vi "fuzzyex Set Move Direction.vi"(1 "方向":bool, 2 "beta":dbl format="%.2f", 3 "y(VC)":dbl format="%.2f", 4 "x(VC)":dbl format="%.2f") -> (0 "新建目录":bool)   [LabVIEW 2018]
doc: "本VI根据车辆中心坐标、车辆方位角和当前移动方向，在车辆驱动控制范例中计算适当的移动方向。如果车辆不能向后移动到其最终位置，则前进，获得足够的空间后再后退。"
panel:
  # "车辆中心的X坐标"
  # "前进行驶"
  # "车辆中心的Y坐标"
  # "后退行驶"
  # "车辆方位角"
  # "前进行驶"
  # "后退行驶"
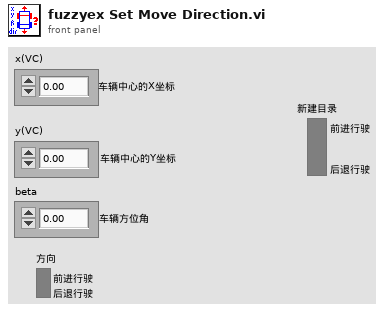
[diagram p1: front panel]
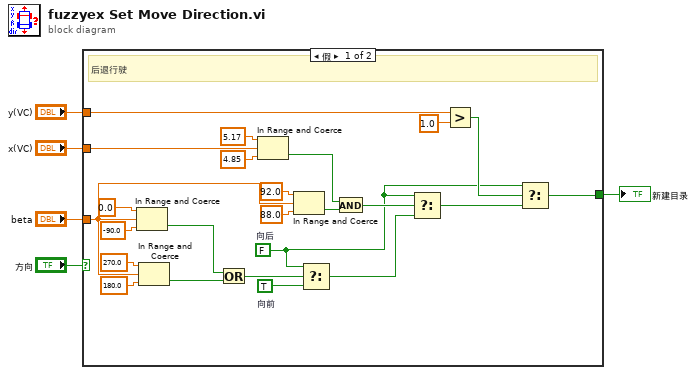
[diagram p0: block diagram]
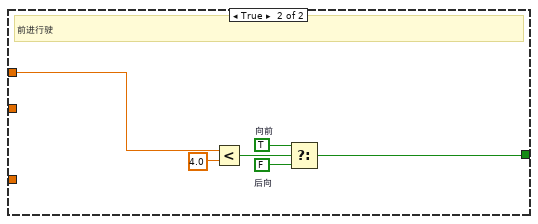
[diagram p2: hidden frame]
diagram:
  n1 = case shown="假" "方向" {
    tunnel: "x(VC)" -> [w27 _]
    tunnel: "y(VC)" -> [w8 w35]
    tunnel: "beta" -> [w13 _]
    tunnel: [w19 w30] -> w1
    frame False {
      w6 = FALSE  # 向后
      w9 = TRUE  # 向前
      # "后退行驶"
      n2 = In Range and Coerce(upper limit=0.0, x=w13, lower limit=-90.0) -> (In Range?=w12:bool)  [unwired: 1 out]
      n3 = In Range and Coerce(upper limit=270.0, x=w13, lower limit=180.0) -> (In Range?=w11:bool)  [unwired: 1 out]
      n4 = Or(x=w12, y=w11) -> (x .or. y?=w7:bool)
      n5 = In Range and Coerce(upper limit=5.17, x=w27, lower limit=4.85) -> (In Range?=w22:bool)  [unwired: 1 out]
      n6 = In Range and Coerce(upper limit=92.0, x=w13, lower limit=88.0) -> (In Range?=w18:bool)  [unwired: 1 out]
      n7 = Select(t=w6, s=w7, f=w9) -> (s? t:f=w10:bool)
      n8 = And(x=w22, y=w18) -> (x .and. y?=w21:bool)
      n9 = Select(t=w6, s=w21, f=w10) -> (s? t:f=w20:bool)
      n10 = Greater?(x=w8, y=1.0) -> (0:w28:bool)
      n11 = Select(t=w6, s=w28, f=w20) -> (s? t:f=w19:bool)
    }
    frame True {
      w31 = FALSE  # 后向
      w32 = TRUE  # 向前
      # "前进行驶"
      n12 = Less?(x=w35, y=4.0) -> (x < y?=w33:bool)
      n13 = Select(t=w32, s=w33, f=w31) -> (s? t:f=w30:bool)
    }
  }
  "新建目录" <- w1
